vi "Write PV URL.vi"(8 "error in (no error)":errorcluster, 10 "PV URL":string, 11 "PV in":refnum<class "PV.lvclass">) -> (0 "error out":errorcluster, 3 "PV out":refnum<class "PV.lvclass">)   [LabVIEW 2015, in "CS++ProcessVariables.lvlib" / "PV.lvclass"]
doc: "Write PV URL."
uses:
  PV.lvclass
  PV.lvclass/PV.ctl
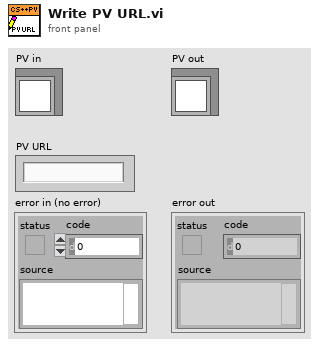
[diagram p1: front panel]
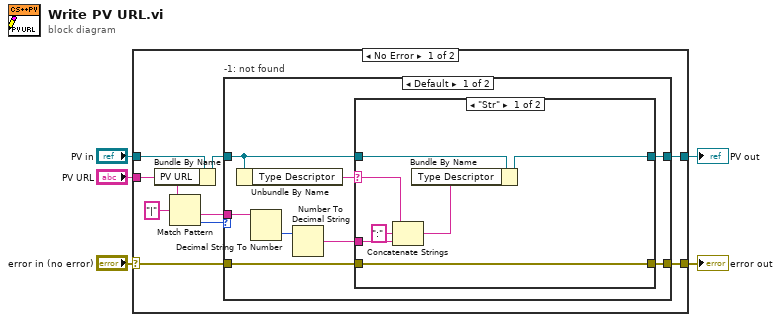
[diagram p0: block diagram]
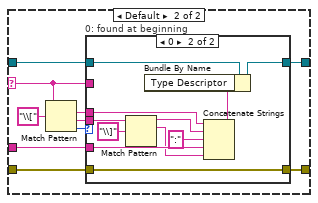
[diagram p2: hidden frame]
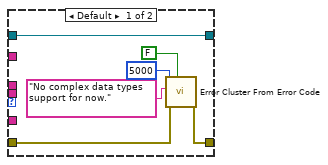
[diagram p3: hidden frame]
diagram:
  n1 = case shown="No Error" "error in (no error)" {
    selector: "error in (no error)" -> [w7 w59]
    tunnel: [w6 w59] -> w4
    tunnel: [w14 w60] -> w2
    tunnel: "PV in" -> [w13 w60]
    tunnel: "PV URL" -> [w9 _]
    frame No Error {
      n2 = Bundle By Name(cluster=w13, "PV URL"=w9) -> (w12:refnum<class "PV.lvclass">)
      n3 = Match Pattern(string=w9, regular expression="|") -> (after substring=w10:string, offset past match=w11:i32)  [unwired: 1 in, 2 out]
      n4 = case "-1: not found" shown="Default" w11 {
        tunnel: [w22 w58] -> w14
        tunnel: w12 -> [w21 w58]
        tunnel: w10 -> [w18 _]
        tunnel: w7 -> [w16 w57]
        tunnel: [w15 w57] -> w6
        frame Default {
          n5 = Unbundle By Name(w21) -> ("Type Descriptor"=w20:string)
          n6 = Decimal String To Number(string=w18) -> (number=w19:i32)  [unwired: 2 in, 1 out]
          n7 = Number To Decimal String(number=w19) -> (decimal integer string=w17:string)  [unwired: 1 in]
          n8 = case shown="\"Str\"" w20 {
            selector: w20 -> [w27 w36]
            tunnel: [w29 w39] -> w22
            tunnel: w21 -> [w28 w38]
            tunnel: w17 -> [w25 w37]
            tunnel: w16 -> [w24 w31]
            tunnel: [w24 w30] -> w15
            frame "Str" {
              n9 = Concatenate Strings(w27, ":" ("string"), w25) -> (w26:string)
              n10 = Bundle By Name(cluster=w28, "Type Descriptor"=w26) -> (w29:refnum<class "PV.lvclass">)
            }
            frame Default {
              n11 = Match Pattern(string=w36, regular expression="\\[") -> (match substring=w32:string, after substring=w33:string, offset past match=w35:i32)  [unwired: 1 in, 1 out]
              n12 = case "0: found at beginning" shown="0" w35 {
                tunnel: [w45 w56] -> w39
                tunnel: w38 -> [w45 w55]
                tunnel: w36 -> [_ _]
                tunnel: w37 -> [_ w53]
                tunnel: w33 -> [_ w51]
                tunnel: w32 -> [_ w50]
                tunnel: w31 -> [w42 w46]
                tunnel: [w41 w46] -> w30
                frame Default {
                  n13 = call <vilib>:"Error Cluster From Error Code.vi"("show call chain? (False)"=FALSE, "error in (no error)"=w42, "error message (\"\")"="No complex data types support for now." ("error message (\"\")"), "error code (0)"=5000) -> ("error out"=w41:errorcluster)  [unwired: 5 in]
                }
                frame 0 {
                  n14 = Match Pattern(string=w51, regular expression="\\]") -> (before substring=w49:string, match substring=w47:string)  [unwired: 1 in, 2 out]
                  n15 = Concatenate Strings(w50, w49, ":" ("string"), w53, w47) -> (w54:string)
                  n16 = Bundle By Name(cluster=w55, "Type Descriptor"=w54) -> (w56:refnum<class "PV.lvclass">)
                }
              }
            }
          }
        }
        frame -1 {
        }
      }
    }
    frame Error {
    }
  }
  "error out" <- w4
  "PV out" <- w2
